vi "VIChallenge Main.vi"() -> ()   [LabVIEW 2013, in "VIChallenge.lvlib"]
uses:
  VIChallenge.lvlib
  Worker State.ctl
  <vilib>/LabVIEW Hacker/LVH-Toolbox/Common/LVH-Common.lvlib
  <vilib>/National Instruments/LabVIEW Interface for Amazon S3/LV Interface for Amazon S3.lvlib
panel:
  out "Iterations":i32
  in  "Stop Button":bool
  out "Error Out":errorcluster
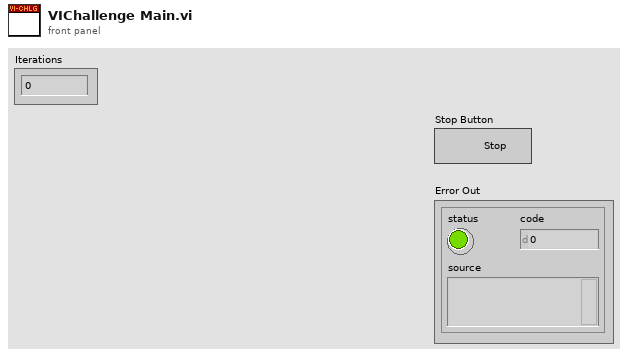
[diagram p1: front panel]
types:
  T1 = typedef "VIChallenge.lvlib/Worker State.ctl" = enum16{"Poll For Job", "Get Source", "Grade", "Upload Results", "Notify User"}
  T2 = typedef "VIChallenge.lvlib/VIChallenge Config.ctl" = cluster{"AWS Credentials":T3, "AWS Account Number":string, "SQS Jobs":refnum<class "AWS_SQS.lvclass">, "SQS Status":refnum<class "AWS_SQS.lvclass">, "Source Dir":path, "Working Dir":path, "Output Dir":path, "Archive Dir":path, "job":T4}
  T3 = typedef "AWS_Core.lvlib/AWS_AWS Credentials.ctl" = cluster{"AWSAccessKeyId":string, "Secret Key":string}
  T4 = typedef "VIChallenge.lvlib/JSON_job.ctl" = cluster{"job_id":string, "challenge_id":string, "user_id":string, "s3_source_bucket":string, "s3_source_directory":string, "s3_source_filename":string, "status_queue_name":string}
  T5 = enum16{"open", "replace", "create", "open or create", "replace or create", "replace or create with confirmation"}
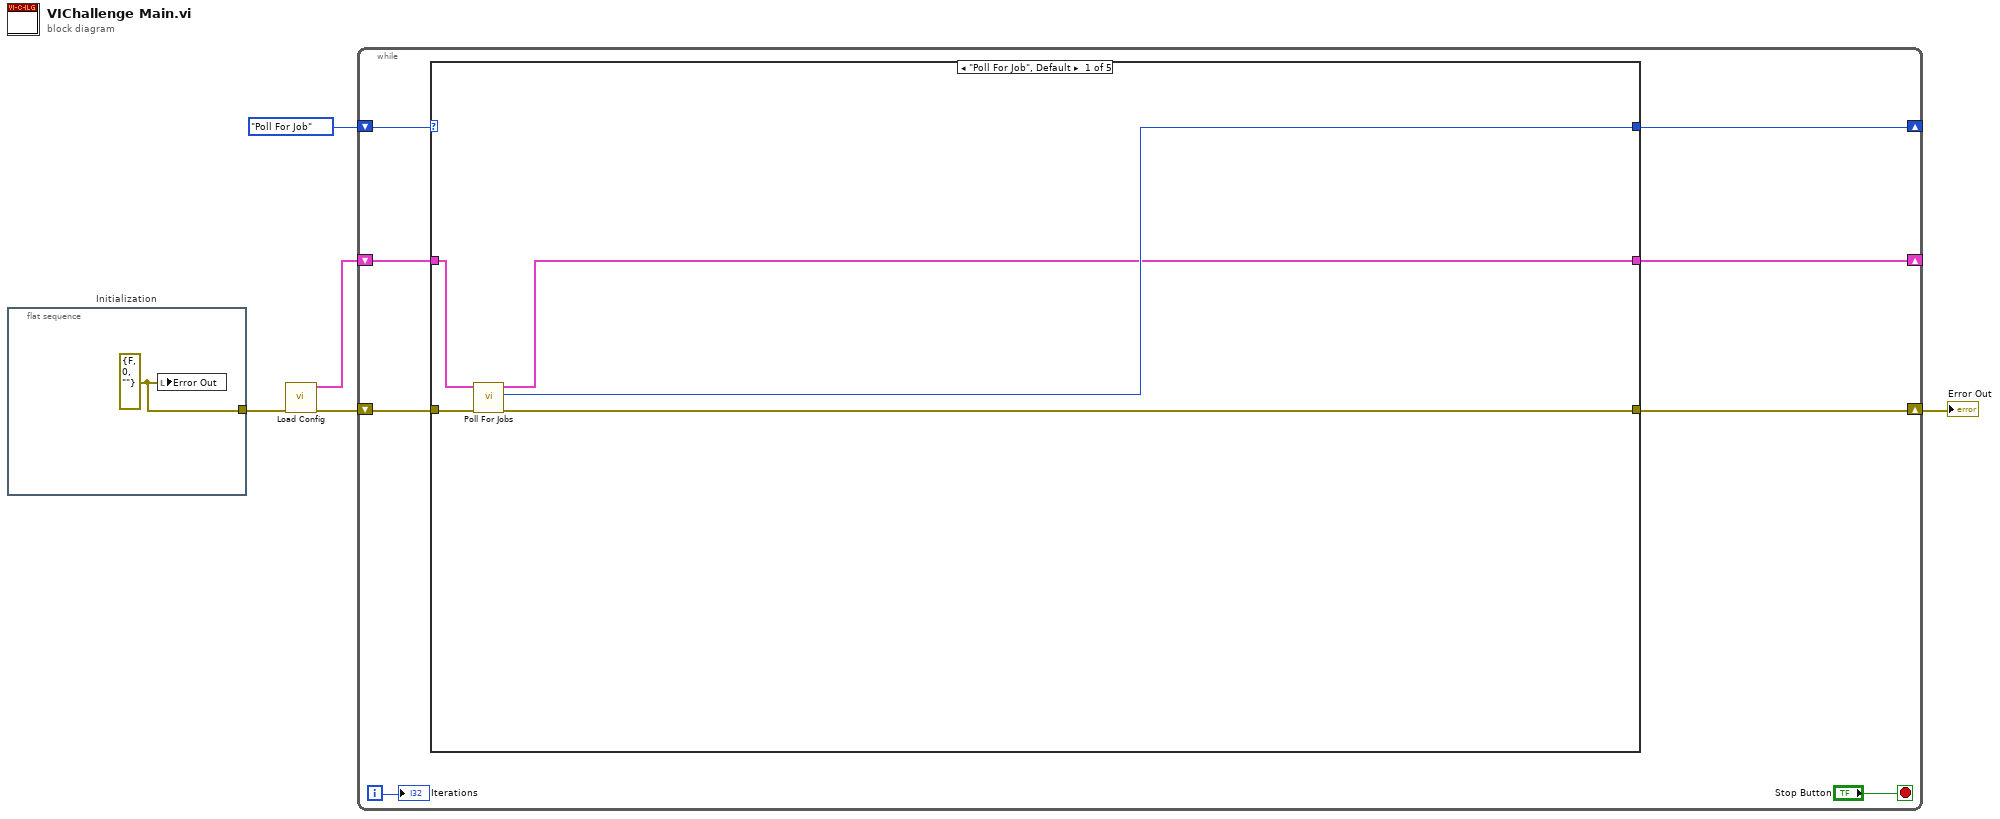
[diagram p0: block diagram]
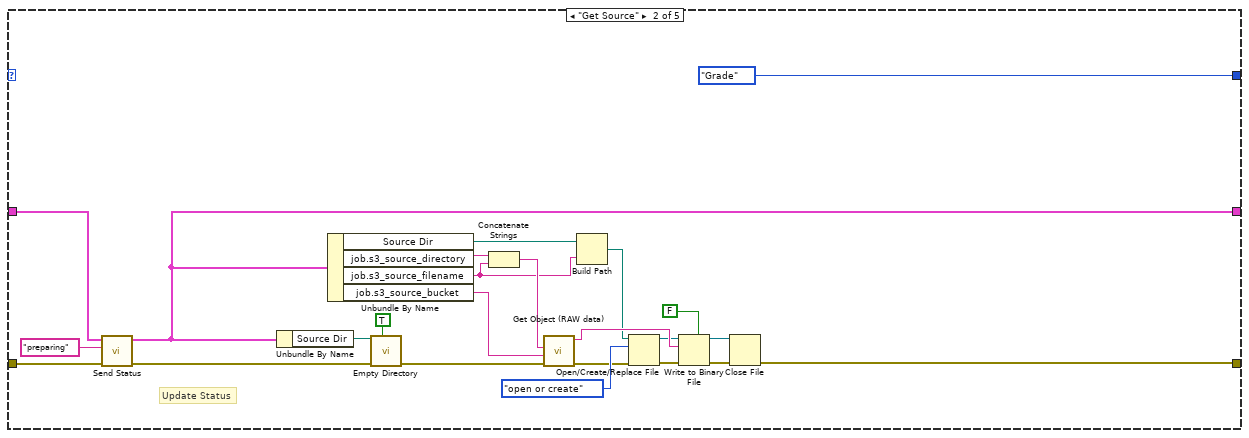
[diagram p2: hidden frame]
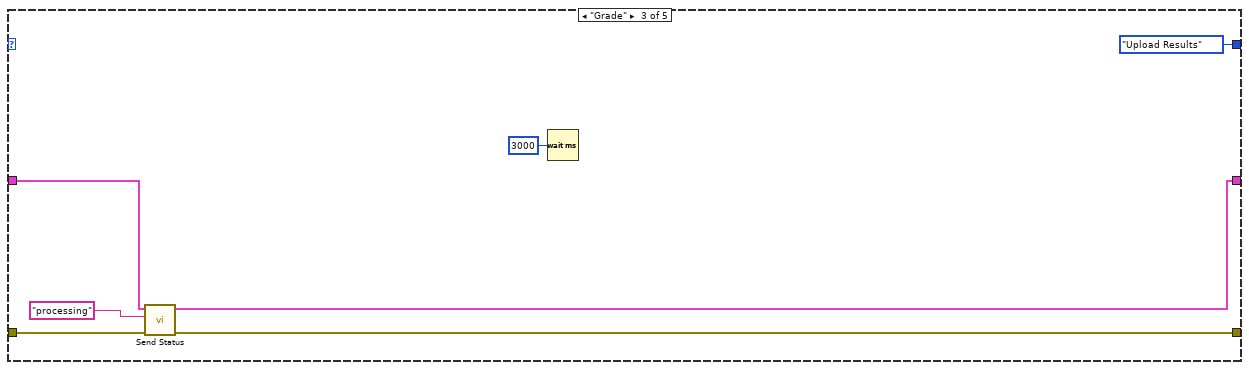
[diagram p3: hidden frame]
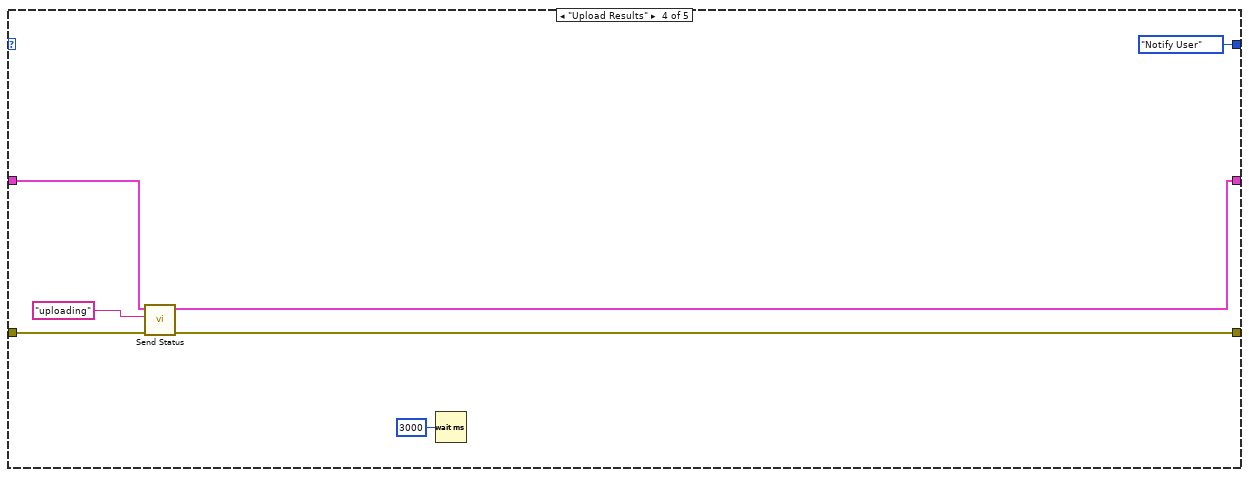
[diagram p4: hidden frame]
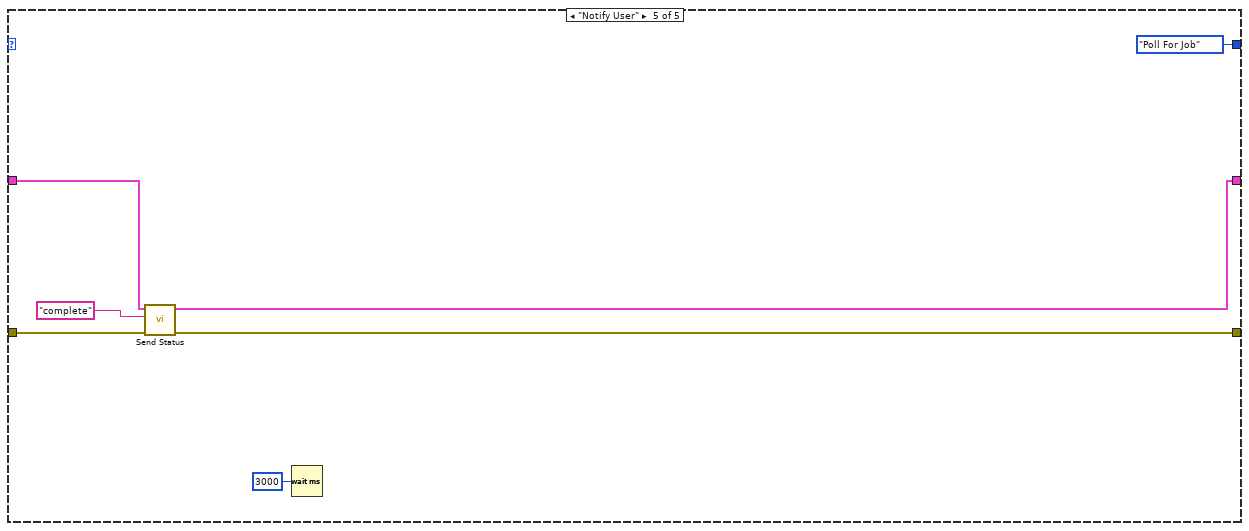
[diagram p5: hidden frame]
diagram:
  n1 = flat-sequence "Initialization" {
    tunnel: [w6] -> w3
    frame #0 {
      w6 = errorcluster {"status"=FALSE, "code"=0, "source"=""} ("Error Out")
      n2 = local write "Error Out"(w6) -> ()
    }
  }
  n3 = call "Load Config.vi"("Error In"=w3) -> ("Error Out"=w2:errorcluster, "VIChallenge Config"=w1:T2)  [unwired: 9 in]
  n4 = while {
    shift-right: [w12] -> w4
    shift-left: w2 -> [w13]
    shift-right: [w7] -> _
    shift-left: Worker_State."Poll For Job" ("Worker State") -> [w14]
    shift-right: [w10] -> _
    shift-left: w1 -> [w11]
    i -> [w8]
    stop <- "Stop Button" stop-if-true
    n5 = case shown="\"Poll For Job\", Default" w14 {
      tunnel: w13 -> [w19 w23 w49 w56 w63]
      tunnel: [w18 w26 w48 w55 w62] -> w12
      tunnel: w11 -> [w17 w22 w47 w54 w61]
      tunnel: [w15 w21 w46 w53 w60] -> w10
      tunnel: [w16 Worker_State."Grade" ("Worker State") Worker_State."Upload Results" ("Worker State") Worker_State."Notify User" ("Worker State") Worker_State."Poll For Job" ("Worker State")] -> w7
      frame "Poll For Job", Default {
        n6 = call "Poll For Jobs.vi"("Error In"=w19, "VIChallenge Config in"=w17) -> ("Error Ou"=w18:errorcluster, "Worker State"=w16:T1, "VIChallenge Config out"=w15:T2)  [unwired: 7 in]
      }
      frame "Get Source" {
        # "Update Status"
        n7 = call "Send Status.vi"("Error In"=w23, "Status"="preparing", "VIChallenge Config"=w22) -> ("Error Out"=w24:errorcluster, "VIChallenge Config"=w21:T2)  [unwired: 7 in]
        n8 = Unbundle By Name(w21) -> ("Source Dir"=w42:path)
        n9 = Unbundle By Name(w21) -> ("Source Dir"=w28:path, "job.s3_source_directory"=w30:string, "job.s3_source_filename"=w27:string, "job.s3_source_bucket"=w31:string)
        n10 = call <vilib>:"Empty Directory.vi"("Delete Files Without Prompt? (F)"=TRUE, "Error In"=w24, "Directory"=w42) -> ("Error Out"=w32:errorcluster)  [unwired: 6 in, 2 out]
        n11 = Concatenate Strings(w30, w27) -> (w29:string)
        n12 = call <vilib>:"Get Object (RAW data).vi"("error in (no error)"=w32, "Bucket"=w31, "Path"=w29) -> ("error out"=w35:errorcluster, "Data"=w39:string)  [unwired: 6 in, 1 out]
        n13 = Build Path(base path=w28, name or relative path=w27) -> (appended path=w36:path)
        n14 = Open/Create/Replace File(file path (use dialog)=w36, error in=w35, operation (0:open)=T5."open or create") -> (refnum out=w37:refnum<file>, error out=w33:errorcluster)  [unwired: 3 in, 1 out]
        n15 = Write to Binary File(file (use dialog)=w37, data=w39, error in=w33, 5:FALSE ("prepend array or string size? (T)")) -> (refnum out=w38:refnum<file>, error out=w34:errorcluster)  [unwired: 2 in, 1 out]
        n16 = Close File(refnum=w38, error in=w34) -> (error out=w26:errorcluster)  [unwired: 1 out]
      }
      frame "Grade" {
        n17 = call "Send Status.vi"("Error In"=w49, "Status"="processing", "VIChallenge Config"=w47) -> ("Error Out"=w48:errorcluster, "VIChallenge Config"=w46:T2)  [unwired: 7 in]
        n18 = Wait (ms)(milliseconds to wait=u32 3000) -> ()  [unwired: 1 out]
      }
      frame "Upload Results" {
        n19 = call "Send Status.vi"("Error In"=w56, "Status"="uploading", "VIChallenge Config"=w54) -> ("Error Out"=w55:errorcluster, "VIChallenge Config"=w53:T2)  [unwired: 7 in]
        n20 = Wait (ms)(milliseconds to wait=u32 3000) -> ()  [unwired: 1 out]
      }
      frame "Notify User" {
        n21 = call "Send Status.vi"("Error In"=w63, "Status"="complete", "VIChallenge Config"=w61) -> ("Error Out"=w62:errorcluster, "VIChallenge Config"=w60:T2)  [unwired: 7 in]
        n22 = Wait (ms)(milliseconds to wait=u32 3000) -> ()  [unwired: 1 out]
      }
    }
    "Iterations" <- w8
  }
  "Error Out" <- w4
